vi "Gyro_Angle.vi"(8 "Mod":dbl, 11 "Input":dbl) -> (3 "Output":dbl)   [LabVIEW 2016]
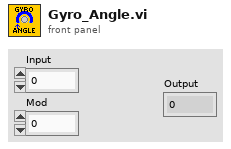
[diagram p1: front panel]
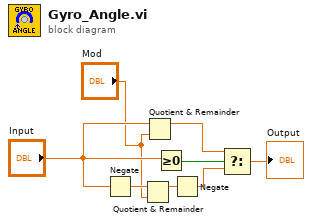
[diagram p0: block diagram]
diagram:
  n1 = Negate(x="Input") -> (-x=w7:dbl)
  n2 = Quotient & Remainder(x=w7, y="Mod") -> (x-y*floor(x/y)=w8:dbl)  [unwired: 1 out]
  n3 = Quotient & Remainder(x="Input", y="Mod") -> (x-y*floor(x/y)=w5:dbl)  [unwired: 1 out]
  n4 = Greater Or Equal To 0?(x="Input") -> (x >= 0?=w6:bool)
  n5 = Negate(x=w8) -> (-x=w4:dbl)
  n6 = Select(t=w5, s=w6, f=w4) -> (s? t:f=→"Output":dbl)
